vi "Release Sequence File.vi"(7 "SequenceFile":refnum<k7>, 8 "error in (no error)":errorcluster, 11 "Session Handle in":T1) -> (0 "error out":errorcluster, 3 "Session Handle out":T1)   [LabVIEW 2019, in "HTS.lvlib" / "Engine.lvclass"]
uses:
  Engine/Engine.lvclass
  Engine/Typedefs/Session Handle.ctl
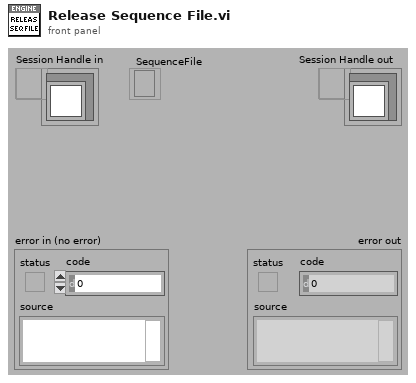
[diagram p1: front panel]
types:
  T1 = typedef "HTS.lvlib/Engine.lvclass/Session Handle.ctl" = refnum<data-value>
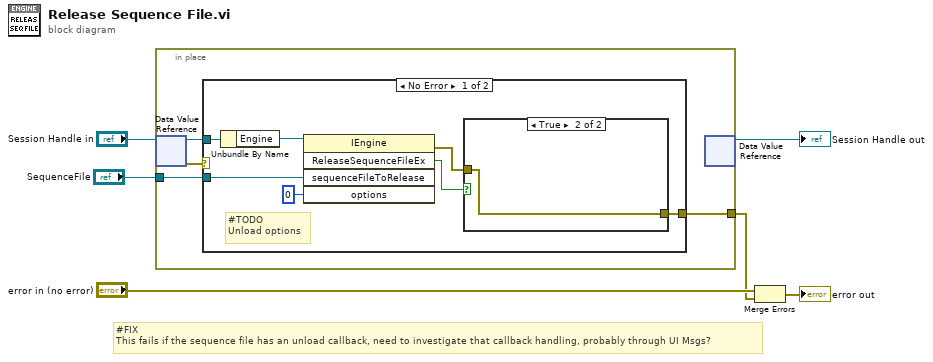
[diagram p0: block diagram]
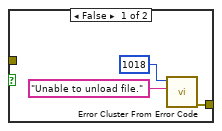
[diagram p2: hidden frame]
diagram:
  # "#FIX\nThis fails if the sequence file has an unload callback, need to investigate that callback handling, probably through UI Msgs?"
  n1 = in-place {
    in-place-border: "SequenceFile" -> [w8]
    in-place-border: [w7] -> w1
    n2 = in-place-dvr #1("Session Handle in") -> (w9:refnum<class "Engine.lvclass">, w10:errorcluster)
    n3 = case shown="No Error" w10 {
      selector: w10 -> [_ w22]
      tunnel: w9 -> [w17 _]
      tunnel: w8 -> [w15 _]
      tunnel: [w11 w22] -> w7
      frame No Error {
        # "#TODO\nUnload options"
        n4 = Unbundle By Name(w17) -> ("Engine"=w16:refnum<k7>)
        n5 = invoke class="IEngine" method="ReleaseSequenceFileEx"(reference=w16, "sequenceFileToRelease"=w15, "options"=0) -> (error out=w12:errorcluster, "ReleaseSequenceFileEx"=w13:bool)  [unwired: 2 in, 3 out]
        n6 = case shown="True" w13 {
          tunnel: w12 -> [_ w21]
          tunnel: [w18 w21] -> w11
          frame False {
            n7 = call <vilib>:"Error Cluster From Error Code.vi"("error message (\"\")"="Unable to unload file." ("error message (\"\")"), "error code (0)"=1018) -> ("error out"=w18:errorcluster)  [unwired: 7 in]
          }
          frame True {
          }
        }
      }
      frame Error {
      }
    }
    n8 = in-place-dvr #1() -> (→"Session Handle out":T1)  [unwired: 1 in, 1 out]
  }
  n9 = Merge Errors("error in (no error)", w1) -> (→"error out":errorcluster)
